vi "Variant Type is Complex.vi"(8 "error in (no error)":errorcluster, 11 "Type":variant) -> (0 "error out":errorcluster, 3 "Sortable ?":bool)   [LabVIEW 2012, in "Scripting Tools.lvlib" / "XNode Support.lvlib"]
uses:
  XNode Support.lvlib
  <vilib>/Utility/VariantDataType/VariantType.lvlib
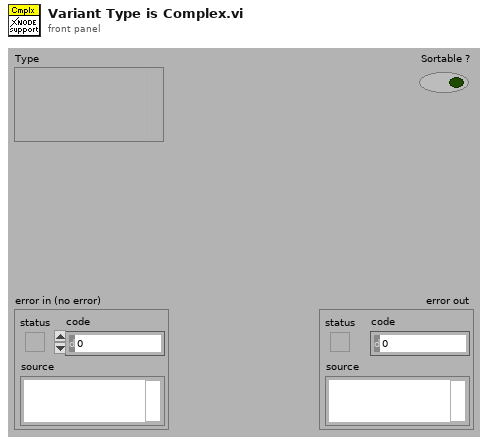
[diagram p1: front panel]
types:
  T1 = typedef "VariantType.lvlib/Type.ctl" = enum8{"Invalid Type", "Void", "I8", "I16", "I32", "I64", "U8", "U16", "U32", "U64", "Single Float", "Double Float", "Extended Float", "Single Complex", "Double Complex", "Extended Complex", "Enum U8", "Enum U16", "Enum U32", "Enum U64", "Single Float With Unit", "Double Float With Unit", "Extended Float With Unit", "Single Complex with Unit", "Double Complex with Unit", "Extended Complex with Unit", "Boolean", "String", "Path", "Picture", "Tag", "Array", "Cluster", "Variant", "LV Variant", "Waveform", "Timestamp", "Digital Waveform", "Digital Data", "ExpressData", "Refnum", "External Data", "VI", "Poly VI", "LabVIEW Class Instance", "Fixed Point"}
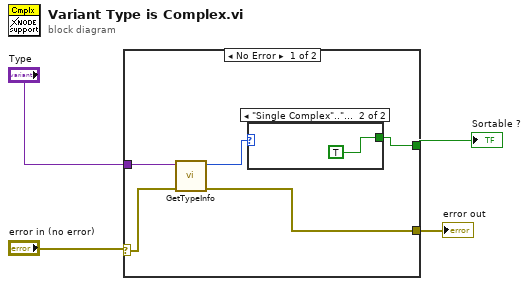
[diagram p0: block diagram]
diagram:
  n1 = case shown="No Error" "error in (no error)" {
    selector: "error in (no error)" -> [w7 w11]
    tunnel: "Type" -> [w9 _]
    tunnel: [w8 w11] -> w3
    tunnel: [w5 _] -> w1
    frame No Error {
      n2 = call <vilib>:"GetTypeInfo.vi"("error in (no error)"=w7, "Variant"=w9) -> ("error out"=w8:errorcluster, "Type Enum"=w6:T1)  [unwired: 8 out]
      n3 = case shown="\"Single Complex\"..\"Extended Complex\", \"Single Complex with Unit\"..\"Extended Complex with Unit\"" w6 {
        tunnel: [_ TRUE] -> w5
        frame "Invalid Type", Default {
        }
        frame "Single Complex".."Extended Complex", "Single Complex with Unit".."Extended Complex with Unit" {
        }
      }
    }
    frame Error {
    }
  }
  "Sortable ?" <- w1
  "error out" <- w3
